vi "CD Init.vi"(8 "Error (in)":errorcluster, 11 "Device Reference":T14 format="%.0x") -> (0 "Error (out)":errorcluster, 1 "Inline Status Channels Refs":T3[](array[typedef]) format="%.0x", 2 "Card Parameters (out)":T25, 3 "RT Inline Data_Data Description_Channels":T17[](array[typedef]) {"Frame Drescriptors"."RT"."Status Channel Ref" format="%.0x"; "Frame Drescriptors"."RT"."Words Block Data Refs"."Data Reference" format="%.0x"; "Frame Drescriptors"."RT"."Timestamp Channel Data Reference" format="%.0x"; "Frame Drescriptors"."BC"."Status Channel Refs" format="%.0x"; "Frame Drescriptors"."BC"."param block data refs"."Data Reference" format="%.0x"; "Frame Drescriptors"."BC"."Timestamp Channel Data Reference" format="%.0x"}, 6 "RT Async Data":T1 {"Map (MC Tx)"."Word Data Reference" format="%.0x"; "Map (MC Rx)"."Channel Data Reference" format="%.0x"; "Map (RT Command Channels)"."RT Command Channel Ref" format="%.0x"; "MAP (BC Acyclic Messages Trigger)"."Acyclic Message Trigger Channel Ref" format="%.0x"; "Map (Bc Command Channels)"."BC Command Channel Ref" format="%.0x"; "Map (RT to ..)"."Word Data Reference" format="%.0x"; "Map (BC to RT)"."Channel Data Reference" format="%.0x"})   [LabVIEW 2020, in "Ballard MIL-1553 Engine.lvlib"]
doc: "This VI reads all properties, creates different Maps (Tx) and initializes the Core of the board using XML file. Initialization is done here because Rx part is done Inline and Tx part asynchronously."
uses:
  Ballard MIL-1553 Engine.lvlib
  <vilib>/NI VeriStand/Custom Device API/Custom Device Item Ref.ctl
  Controls/Card Parameters.ctl
  Shared/Controls and Global/Initialization Method.ctl
  Controls/RT Inline Data_Data Description_Channel.ctl
  Controls/RT Inline Frame Descriptor.ctl
  Controls/RT Inline Frame Descriptor_BC.ctl
  <vilib>/NI VeriStand/Custom Device API/Data Reference.ctl
  <vilib>/NI VeriStand/Custom Device API/Block Data Reference.ctl
  Shared/EncodeDecode/_typedefs/parameter_config_type.ctl
  Shared/EncodeDecode/_typedefs/parameter_config_type_type.ctl
  Shared/EncodeDecode/_typedefs/parameter_config_encoding_type.ctl
  Controls/RT Inline Frame Descriptor_RT.ctl
  Shared/Controls and Global/RT CWD2.ctl
  Shared/Controls and Global/RT CWD1.ctl
  Shared/Controls and Global/RT messageType.ctl
  Controls/RT Async Data.ctl
  Controls/RT Async_Map BC2RT.ctl
  Controls/RT Async_Map_Type.ctl
  Controls/RT Async_Raw Values.ctl
  Controls/RT Async_Raw Values to Messages Index_Association.ctl
  Controls/Asynchronous - Parameter map_type.ctl
  Controls/RT Async_Map RT2BC.ctl
  Controls/RT Async_Map RTs Status.ctl
  Controls/RT Async_Map BC Command Channels.ctl
  Controls/RT Async_Map BC Acyclic Messages Trigger.ctl
  Controls/RT Async_Map RT Command Channels.ctl
  Controls/RT Init States.ctl
  Shared/Controls and Global/Compiled.Settings.ctl
  Shared/Controls and Global/RT Channel.ctl
  Shared/Controls and Global/RT BC.ctl
  Shared/Controls and Global/RT Message.ctl
  Shared/Controls and Global/RT Remote Terminal.ctl
  Shared/Controls and Global/RT Remote Terminal_rtMode.ctl
  Shared/Controls and Global/RT Remote Terminal_RT subAddress.ctl
  Shared/Controls and Global/RT Remote Terminal_RT direction.ctl
  Shared/Controls and Global/RT Remote Terminal_RT Mode Code.ctl
  a0ee2a4f-e665-4580-bc02-68e9c6553bf0.vi
  abe306a3-0000-4c3f-84a0-3b77fc310cf4.vi
  Shared/Controls and Global/Global.vi
  <vilib>/NI VeriStand/Custom Device API/Get Item Property (I32).vi
  <vilib>/NI VeriStand/Custom Device API/Get Item Property (U16).vi
  <vilib>/NI VeriStand/Custom Device API/Get Item Property (Variant).vi
  <vilib>/JDP Science/JSONtext/Variant to JSON Text.vi
  <vilib>/NI VeriStand/Custom Device API/Custom Device API.lvlib
  <vilib>/NI VeriStand/Custom Device Tools/Custom Device Utility Library/Custom Device Utility Library.lvlib
  Shared/Ballard 1553 Shared.lvlib
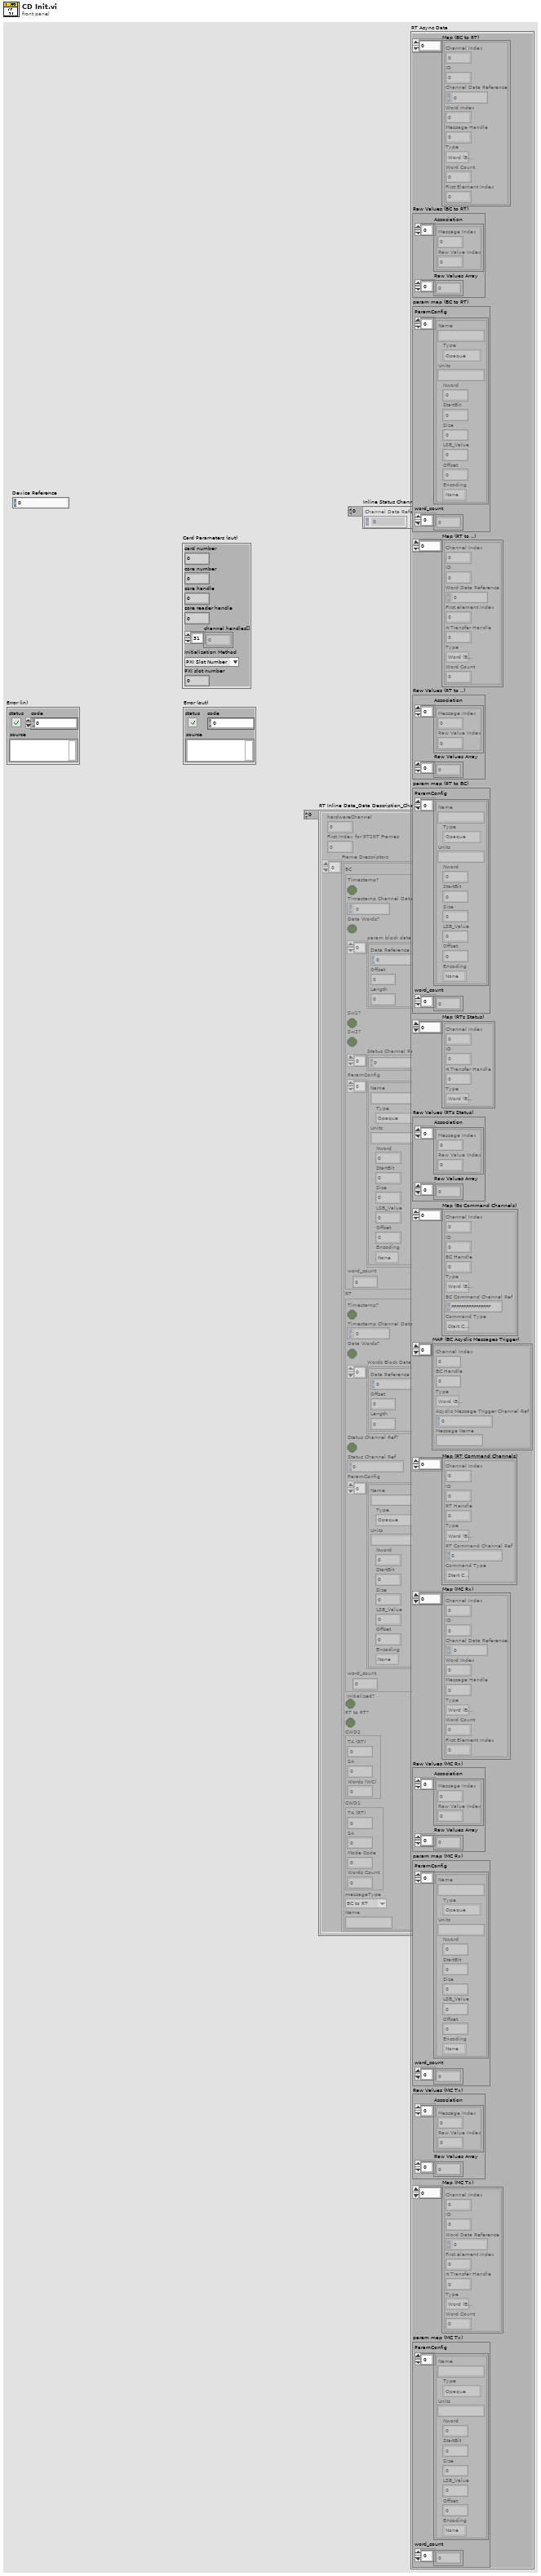
[diagram p1: front panel]
types:
  T1 = typedef "Ballard MIL-1553 Engine.lvlib/RT Async Data.ctl" = cluster{"Map (BC to RT)":T2[], "Raw Values (BC to RT)":T5, "param map (BC to RT)":T7, "Map (RT to ..)":T11[], "Raw Values (RT to ..)":T5, "param map (RT to BC)":T7, "Map (RTs Status)":T12[], "Raw Values (RTs Status)":T5, "Map (Bc Command Channels)":T13[], "MAP (BC Acyclic Messages Trigger)":T15[], "Map (RT Command Channels)":T16[], "Map (MC Rx)":T2[], "Raw Values (MC Rx)":T5, "param map (MC Rx)":T7, "Raw Values (MC Tx)":T5, "Map (MC Tx)":T11[], "param map (MC Tx)":T7}
  T2 = typedef "Ballard MIL-1553 Engine.lvlib/RT Async_Map BC2RT.ctl" = cluster{"Channel Index":i32, "ID":i32, "Channel Data Reference":T3, "Word Index":i32, "Message Handle":u64, "Type":T4, "Word Count":i32, "First Element Index":i32}
  T3 = typedef "Custom Device API.lvlib/Data Reference.ctl" = i32
  T4 = typedef "Ballard MIL-1553 Engine.lvlib/RT Async_Map_Type.ctl" = enum16{"Word (BC to RT)", "Word (MC (Rx))", "Acyclic Message Trigger", "Word (RT to ..)", "Word (RT to RT)", "Word (MC (Tx))", "RT Status", "BC Commands", "RT Commands"}
  T5 = typedef "Ballard MIL-1553 Engine.lvlib/RT Async_Raw Values.ctl" = cluster{"Association":T6[], "Raw Values Array":u16[]}
  T6 = typedef "Ballard MIL-1553 Engine.lvlib/RT Async_Raw Values to Messages Index_Association.ctl" = cluster{"Message Index":i32, "Raw Value Index":i32}
  T7 = typedef "Ballard MIL-1553 Engine.lvlib/Asynchronous - Parameter map_type.ctl" = cluster{"ParamConfig":T8[], "word_count":u8[]}
  T8 = typedef "parameter_config_type.ctl" = cluster{"Name":string, "Type":T9, "Units":string, "Nword":i32, "StartBit":i32, "Size":i32, "LSB_Value":i32, "Offset":i32, "Encoding":T10}
  T9 = typedef "parameter_config_type_type.ctl" = enum16{"Opaque", "Enum", "Float", "Integer", "Bcd", "Bool"}
  T10 = typedef "parameter_config_encoding_type.ctl" = enum16{"None", "2-complement", "Unsigned"}
  T11 = typedef "Ballard MIL-1553 Engine.lvlib/RT Async_Map RT2BC.ctl" = cluster{"Channel Index":i32, "ID":i32, "Word Data Reference":T3, "First element Index":i32, "rt Transfer Handle":u64, "Type":T4, "Word Count":i32}
  T12 = typedef "Ballard MIL-1553 Engine.lvlib/RT Async_Map RTs Status.ctl" = cluster{"Channel Index":i32, "ID":i32, "rt Transfer Handle":u64, "Type":T4}
  T13 = typedef "Ballard MIL-1553 Engine.lvlib/RT Async_Map BC Command Channels.ctl" = cluster{"Channel Index":i32, "ID":i32, "BC Handle":u64, "Type":T4, "BC Command Channel Ref":T14, "Command Type":enum16{"Start Command", "Stop Command"}}
  T14 = typedef "Custom Device API.lvlib/Custom Device Item Ref.ctl" = u64
  T15 = typedef "Ballard MIL-1553 Engine.lvlib/RT Async_Map BC Acyclic Messages Trigger.ctl" = cluster{"Channel Index":i32, "BC Handle":u64, "Type":T4, "Acyclic Message Trigger Channel Ref":T14, "Message Name":string}
  T16 = typedef "Ballard MIL-1553 Engine.lvlib/RT Async_Map RT Command Channels.ctl" = cluster{"Channel Index":i32, "ID":i32, "RT Handle":u64, "Type":T4, "RT Command Channel Ref":T14, "Command Type":enum16{"Start Command", "Stop Command"}}
  T17 = typedef "Ballard MIL-1553 Engine.lvlib/RT Inline Data_Data Description_Channel.ctl" = cluster{"hardwareChannel":u16, "First Index for RT2RT Frames":i32, "Frame Drescriptors":T18[]}
  T18 = typedef "Ballard MIL-1553 Engine.lvlib/RT Inline Frame Descriptor.ctl" = cluster{"BC":T19, "RT":T21, "Initialized?":bool, "RT to RT?":bool, "CWD2":T22, "CWD1":T23, "messageType":T24, "Name":string}
  T19 = typedef "Ballard MIL-1553 Engine.lvlib/RT Inline Frame Descriptor_BC.ctl" = cluster{"Timestamp?":bool, "Timestamp Channel Data Reference":T3, "Data Words?":bool, "param block data refs":T20[], "Sw1?":bool, "Sw2?":bool, "Status Channel Refs":T14[], "ParamConfig":T8[], "word_count":u8}
  T20 = typedef "Custom Device API.lvlib/Block Data Reference.ctl" = cluster{"Data Reference":T3, "Offset":u64, "Length":u64}
  T21 = typedef "Ballard MIL-1553 Engine.lvlib/RT Inline Frame Descriptor_RT.ctl" = cluster{"Timestamp?":bool, "Timestamp Channel Data Reference":T3, "Data Words?":bool, "Words Block Data Refs":T20[], "Status Channel Ref?":bool, "Status Channel Ref":T14, "ParamConfig":T8[], "word_count":u8}
  T22 = typedef "Ballard 1553 Shared.lvlib/RT CWD2.ctl" = cluster{"TA (RT)":i8, "SA":i8, "Words (WC)":i8}
  T23 = typedef "Ballard 1553 Shared.lvlib/RT CWD1.ctl" = cluster{"TA (RT)":i8, "SA":i8, "Mode Code":i8, "Words Count":i8}
  T24 = typedef "Ballard 1553 Shared.lvlib/RT messageType.ctl" = enum16{"BC to RT", "RT to BC", "RT to RT", "MC (Rx)", "MC (Tx)"}
  T25 = typedef "Ballard MIL-1553 Engine.lvlib/Card Parameters.ctl" = cluster{"card number":i32, "core number":i32, "core handle":u64, "core reader handle":u64, "channel handles[]":u64[], "Initialization Method":T26, "PXI slot number":i32}
  T26 = typedef "Ballard 1553 Shared.lvlib/Initialization Method.ctl" = enum16{"PXI Slot Number", "Card Number"}
  T27 = typedef "Ballard MIL-1553 Engine.lvlib/RT Init States.ctl" = enum16{"Initialization", "Get Card Settings", "Get Channel Count", "Parse Channels", "Ballard-1553 Initialize", "Get Status Channels Reference", "Exit"}
  T28 = typedef "Ballard 1553 Shared.lvlib/Compiled.Settings.ctl" = cluster{"Name":string, "channels":T29[]}
  T29 = typedef "Ballard 1553 Shared.lvlib/RT Channel.ctl" = cluster{"name":string, "hardWare Channel Number":u16, "BC":T30, "RTs":T32[]}
  T30 = typedef "Ballard 1553 Shared.lvlib/RT BC.ctl" = cluster{"ID":i32, "name":string, "Command Channels Refs":T14[], "messages":T31[], "Acyclic Frames Trigger Channels Refs":T14[], "Acyclic Frames Names":string[]}
  T31 = typedef "Ballard 1553 Shared.lvlib/RT Message.ctl" = cluster{"Name":string, "messageType":T24, "CWD1":T23, "CWD2":T22, "Status Channel Data Refs":T3[], "param item refs":T14[], "param Block Data Refs":T20[], "param Values Array":u16[], "Timestamp Channel Data Reference":T3, "ID":i32, "Timestamp?":bool, "Data Words?":bool, "Status Channel Ref?":bool, "ParamConfig":T8[], "word_count":u8}
  T32 = typedef "Ballard 1553 Shared.lvlib/RT Remote Terminal.ctl" = cluster{"ID":i32, "name":string, "RT Address":i32, "rtMode":T33, "Command Channels Refs":T14[], "Status Channel Data Reference":T3, "subAddresses":T34[], "Mode Codes":T36[]}
  T33 = typedef "Ballard 1553 Shared.lvlib/RT Remote Terminal_rtMode.ctl" = enum16{"Simulate", "Monitor", "Disable"}
  T34 = typedef "Ballard 1553 Shared.lvlib/RT Remote Terminal_RT subAddress.ctl" = cluster{"name":string, "subAddress":i8, "direction":T35, "Timestamp Channel Data Reference":T3, "param value array":u16[], "param blocj data refs":T20[], "param item refs":T14[], "ID":i32, "Timestamp?":bool, "Data Words?":bool, "param config":T8[], "word_count":u8}
  T35 = typedef "Ballard 1553 Shared.lvlib/RT Remote Terminal_RT direction.ctl" = enum16{"Tx", "Rx"}
  T36 = typedef "Ballard 1553 Shared.lvlib/RT Remote Terminal_RT Mode Code.ctl" = cluster{"name":string, "direction":T35, "Timestamp Channel Data Reference":T3, "param values array":u16[], "param block data refs":T20[], "param item refs":T14[], "ID":i32, "Timestamp?":bool, "Data Words?":bool, "Code Number":i32, "param config":T8[], "word_count":u8}
  T37 = typedef "Custom Device API.lvlib/Custom Device File Dependency.ctl" = cluster{"Source":T38, "RT Destination":path, "ForceDownload?":bool, "SupportedTarget":T40, "Version":string}
  T38 = typedef "Custom Device API.lvlib/Path Specification.ctl" = cluster{"Path":path, "Type":T39}
  T39 = typedef "Custom Device API.lvlib/Path Type.ctl" = enum16{"Absolute", "To Base", "To Common Data Dir", "To Application Data Dir"}
  T40 = typedef "Custom Device API.lvlib/Custom Device Supported Target.ctl" = enum16{"All", "PharLap", "VxWorks", "Windows", "Linux_32_ARM", "Linux_x64", "PharLap & Windows", "PharLap & VxWorks", "VxWorks & Windows"}
  T41 = typedef "Custom Device API.lvlib/Custom Device Item Info.ctl" = cluster{"Name":string, "Is Channel":bool, "GUID":string, "Is Waveform":bool}
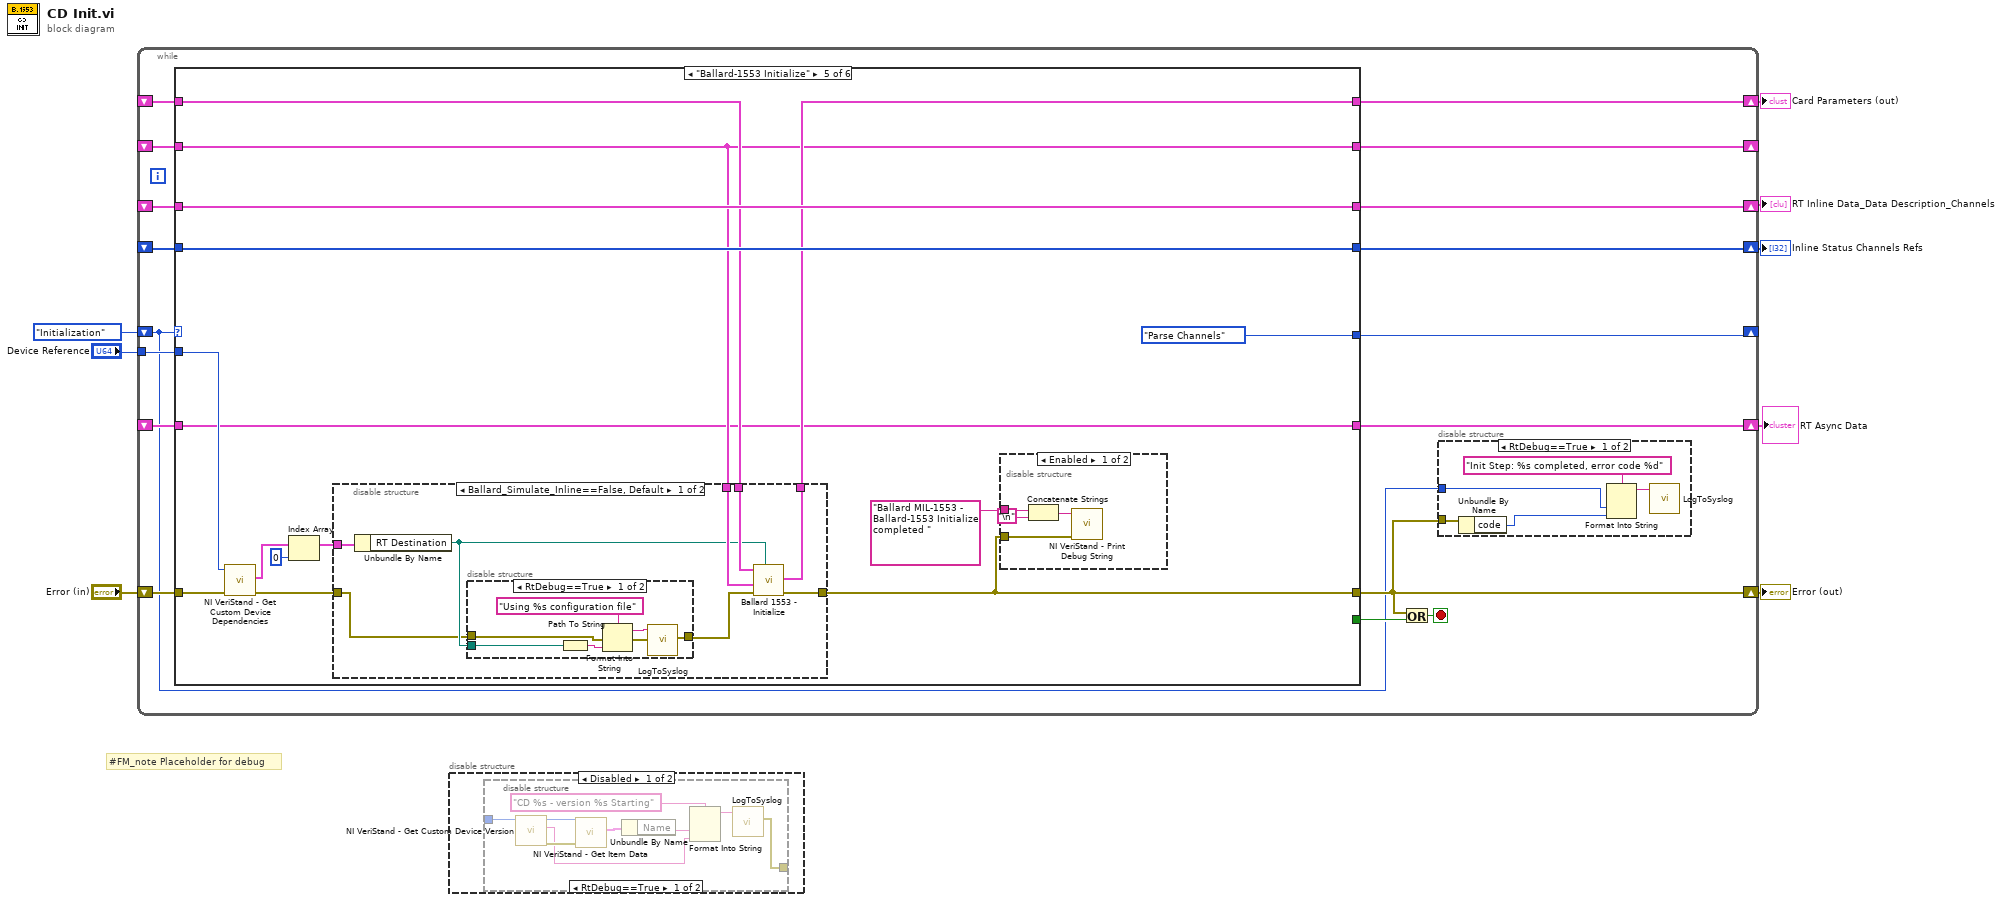
[diagram p0: block diagram]
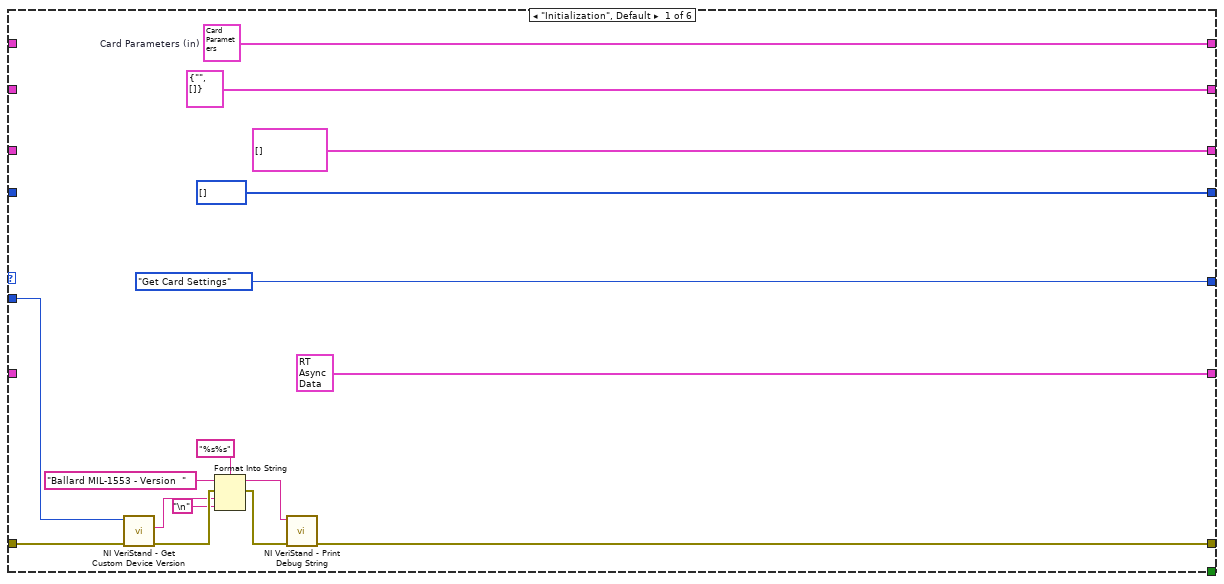
[diagram p5: hidden frame]
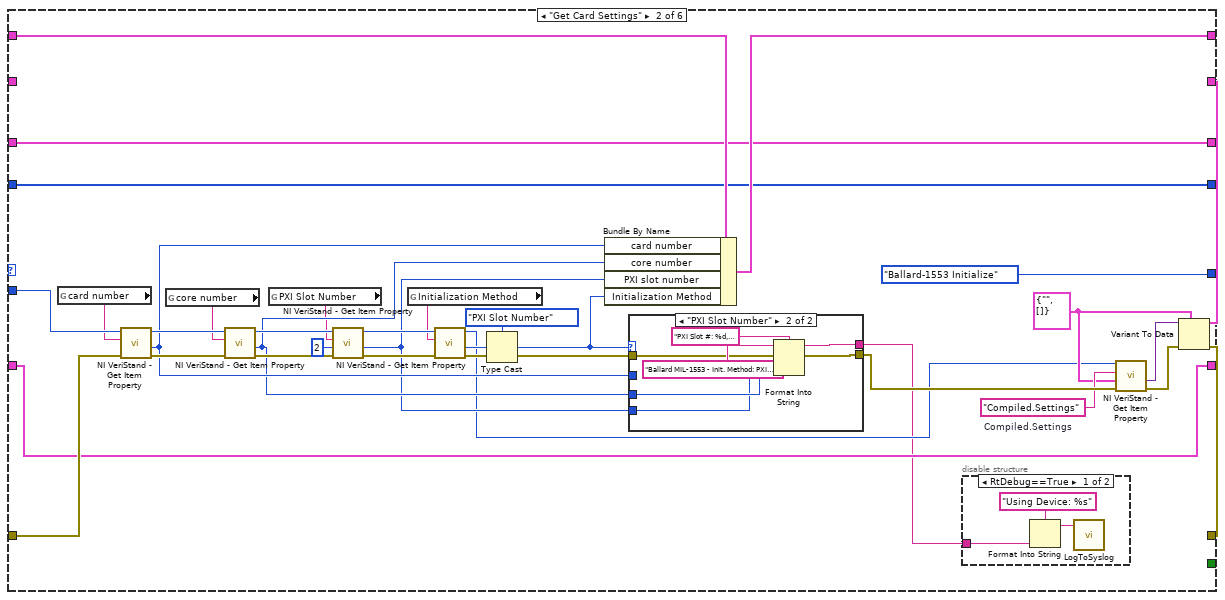
[diagram p6: hidden frame]
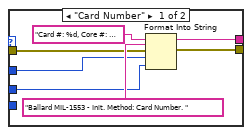
[diagram p8: hidden frame]
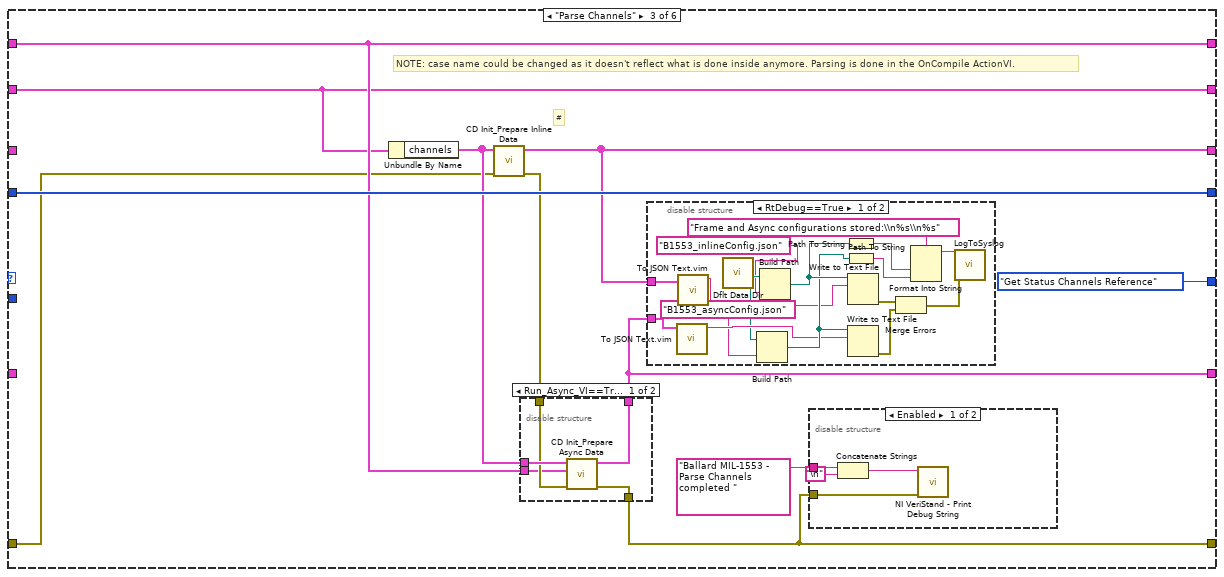
[diagram p9: hidden frame]
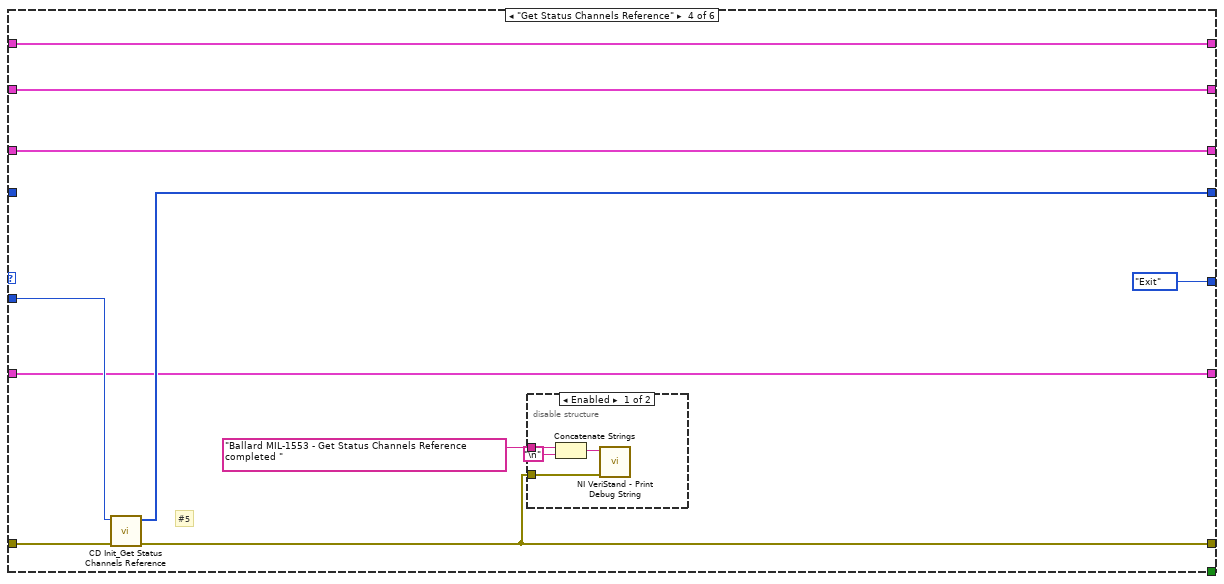
[diagram p13: hidden frame]
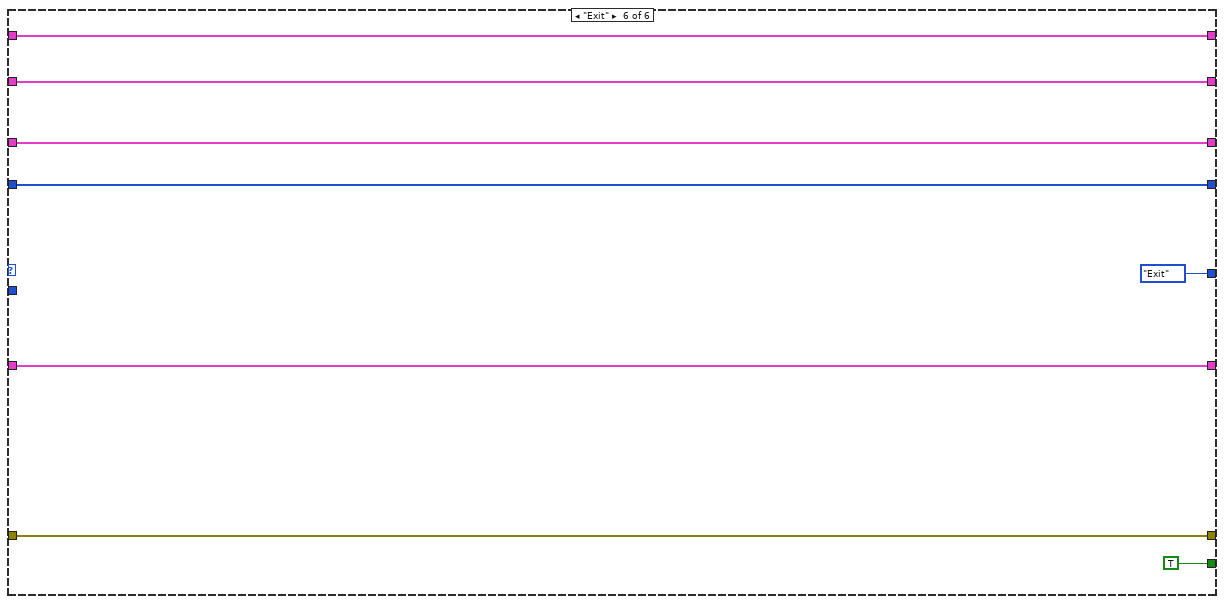
[diagram p18: hidden frame]
diagram:
  # "#FM_note Placeholder for debug"
  n1 = while {
    shift-right: [w11] -> _
    shift-left: RT_Init_States."Initialization" -> [w9]
    tunnel: "Device Reference" -> [w24]
    shift-right: [w20] -> w4
    shift-left: _ -> [w21]
    shift-right: [w19] -> w2
    shift-left: _ -> [w18]
    shift-right: [w17] -> w3
    shift-left: _ -> [w16]
    shift-right: [w10] -> w6
    shift-left: "Error (in)" -> [w25]
    shift-right: [w15] -> _
    shift-left: _ -> [w14]
    shift-right: [w13] -> w1
    shift-left: _ -> [w12]
    stop <- w23 stop-if-true
    n2 = case shown="\"Ballard-1553 Initialize\"" w9 {
      tunnel: w25 -> [w43 w80 w103 w141 w161 w193]
      tunnel: [w41 w49 w101 w136 w150 w193] -> w10
      tunnel: [RT_Init_States."Get Card Settings" RT_Init_States."Ballard-1553 Initialize" RT_Init_States."Get Status Channels Reference" RT_Init_States."Exit" RT_Init_States."Parse Channels" RT_Init_States."Exit"] -> w11
      tunnel: w24 -> [w42 w77 _ w140 w160 _]
      tunnel: [_ _ _ _ _ TRUE] -> w22
      tunnel: w21 -> [_ w76 w106 w142 w154 w190]
      tunnel: [w45 w75 w106 w142 w157 w190] -> w20
      tunnel: [T17[] [] ("RT Inline Data_Data Description_Channels") w74 w100 w145 w159 w189] -> w19
      tunnel: w18 -> [_ w74 _ w145 w159 w189]
      tunnel: [i32[] [] w73 w108 w143 w158 w188] -> w17
      tunnel: w16 -> [_ w73 w108 _ w158 w188]
      tunnel: [T28 {"Name"="", "channels"=[]} ("Compiled.Settings") w48 w104 w139 w153 w187] -> w15
      tunnel: w14 -> [_ _ w104 w139 w153 w187]
      tunnel: [T1 {"Map (BC to RT)"=[], "Raw Values (BC to RT)"={"Association"=[], "Raw Values Array"=[]}, "param map (BC to RT)"={"ParamConfig"=[], "word_count"=[]}, "Map (RT to ..)"=[], "Raw Values (RT to ..)"={"Association"=[], "Raw Values Array"=[]}, "param map (RT to BC)"={"ParamConfig"=[], "word_count"=[]}, "Map (RTs Status)"=[], "Raw Values (RTs Status)"={"Association"=[], "Raw Values Array"=[]}, "Map (Bc Command Channels)"=[], "MAP (BC Acyclic Messages Trigger)"=[], "Map (RT Command Channels)"=[], "Map (MC Rx)"=[], "Raw Values (MC Rx)"={"Association"=[], "Raw Values Array"=[]}, "param map (MC Rx)"={"ParamConfig"=[], "word_count"=[]}, "Raw Values (MC Tx)"={"Association"=[], "Raw Values Array"=[]}, "Map (MC Tx)"=[], "param map (MC Tx)"={"ParamConfig"=[], "word_count"=[]}} ("RT Async Data") w55 w99 w138 w152 w186] -> w13
      tunnel: w12 -> [_ w55 _ w138 w152 w186]
      frame "Initialization", Default {
        w45 = T25 {"card number"=0, "core number"=0, "core handle"=0, "core reader handle"=0, "channel handles[]"=[], "Initialization Method"=enum."PXI Slot Number", "PXI slot number"=0}  # Card Parameters (in)
        n3 = call <vilib>:"NI VeriStand - Get Custom Device Version.vi"("error in (no error)"=w43, "Device Ref in"=w42) -> ("error out"=w40:errorcluster, "Value"=w37:string)  [unwired: 7 in, 1 out]
        n4 = Format Into String(format string="%s%s", initial string="Ballard MIL-1553 - Version  ", error in=w40, w37, "\n") -> (resulting string=w31:string, error out=w39:errorcluster)
        n5 = call <vilib>:"NI VeriStand - Print Debug String.vi"("error in (no error)"=w39, "Message"=w31) -> ("error out"=w41:errorcluster)  [unwired: 9 in]
      }
      frame "Get Card Settings" {
        w52 = "Compiled.Settings"  # Compiled.Settings
        w51 = T28 {"Name"="", "channels"=[]} ("Compiled.Settings")
        n6 = global read "Global.vi" "card number"() -> (w56:string)
        n7 = call-poly <vilib>:"NI VeriStand - Get Item Property.vi"("error in (no error)"=w80, "Property Name"=w56, "Item Ref in"=w77) -> ("error out"=w79:errorcluster, "Value"=w64:i32, "Item Ref out"=w81:T14)  [unwired: 5 in, 1 out]
        n8 = global read "Global.vi" "core number"() -> (w57:string)
        n9 = call-poly <vilib>:"NI VeriStand - Get Item Property.vi"("error in (no error)"=w79, "Property Name"=w57, "Item Ref in"=w81) -> ("error out"=w71:errorcluster, "Value"=w63:i32, "Item Ref out"=w72:T14)  [unwired: 5 in, 1 out]
        n10 = global read "Global.vi" "PXI Slot Number"() -> (w58:string)
        n11 = call-poly <vilib>:"NI VeriStand - Get Item Property.vi"("error in (no error)"=w71, "Default Value"=2, "Property Name"=w58, "Item Ref in"=w72) -> ("error out"=w69:errorcluster, "Value"=w62:i32, "Item Ref out"=w68:T14)  [unwired: 4 in, 1 out]
        n12 = global read "Global.vi" "Initialization Method"() -> (w59:string)
        n13 = call-poly <vilib>:"NI VeriStand - Get Item Property.vi"("error in (no error)"=w69, "Property Name"=w59, "Item Ref in"=w68) -> ("error out"=w61:errorcluster, "Value"=w67:u16, "Item Ref out"=w50:T14)  [unwired: 5 in, 1 out]
        n14 = Type Cast(type=Initialization_Method."PXI Slot Number" ("Initialization Method"), x=w67) -> (*(type *) &x=w65:T26)
        n15 = Bundle By Name(cluster=w76, "card number"=w64, "core number"=w63, "PXI slot number"=w62, "Initialization Method"=w65) -> (w75:T25)
        n16 = case shown="\"PXI Slot Number\"" w65 {
          tunnel: [w91 w98] -> w47
          tunnel: w64 -> [w88 _]
          tunnel: w63 -> [w87 w95]
          tunnel: w62 -> [_ w94]
          tunnel: w61 -> [w86 w93]
          tunnel: [w85 w92] -> w60
          frame "Card Number" {
            n17 = Format Into String(format string="Card #: %d, Core #: %d.", initial string="Ballard MIL-1553 - Init. Method: Card Number. " ("String to write"), error in=w86, w88, w87) -> (resulting string=w91:string, error out=w85:errorcluster)
          }
          frame "PXI Slot Number" {
            n18 = Format Into String(format string="PXI Slot #: %d, Core #: %d.", initial string="Ballard MIL-1553 - Init. Method: PXI Slot Number. " ("String to write"), error in=w93, w94, w95) -> (resulting string=w98:string, error out=w92:errorcluster)
          }
        }
        n19 = disable-structure shown="RtDebug==True" {
          disable-tunnel: w47 -> [w82 _]
          frame condition #0 (active) {
            n20 = Format Into String(format string="Using Device: %s", w82) -> (resulting string=w84:string)  [unwired: 2 in, 1 out]
            n21 = call "LogToSyslog.vi"("message"=w84) -> ()  [unwired: 9 in, 2 out]
          }
          frame condition #1 {
          }
        }
        n22 = call-poly <vilib>:"NI VeriStand - Get Item Property.vi"("error in (no error)"=w60, "Default Value"=w51, "Property Name"=w52, "Item Ref in"=w50) -> ("error out"=w54:errorcluster, "Value"=w53:variant)  [unwired: 4 in, 2 out]
        n23 = Variant To Data(error in=w54, type=w51, Variant=w53) -> (data=w48:T28, error out=w49:errorcluster)
      }
      frame "Parse Channels" {
        # "#"
        # "NOTE: case name could be changed as it doesn't reflect what is done inside anymore. Parsing is done in the OnCompile ActionVI."
        n24 = Unbundle By Name(w104) -> ("channels"=w107:T29[])
        n25 = call "CD Init_Prepare Inline Data.vi"("error in (no error)"=w103, "channels In"=w107) -> ("error out"=w102:errorcluster, "RT Inline Data_Data Description_Channels"=w100:T17[])  [unwired: 8 in]
        n26 = disable-structure shown="Run_Async_VI==True, Default" {
          disable-tunnel: w107 -> [w130 _]
          disable-tunnel: w102 -> [w129 w131]
          disable-tunnel: w106 -> [w128 _]
          disable-tunnel: [w127 _] -> w99
          disable-tunnel: [w126 w131] -> w101
          frame condition #0 (active) {
            n27 = call "CD Init_Prepare Async Data.vi"("error in (no error)"=w129, "Card Parameters (in)"=w128, "Channels In"=w130) -> ("error out"=w126:errorcluster, "RT Async Data"=w127:T1)  [unwired: 7 in]
          }
          frame condition #1 {
          }
        }
        n28 = disable-structure shown="RtDebug==True" {
          disable-tunnel: w100 -> [w117 _]
          disable-tunnel: w99 -> [w116 _]
          frame condition #0 (active) {
            n29 = call "To JSON Text.vim"("Anything"=w116) -> ("<JSON>"=w115:string)  [unwired: 9 in, 1 out]
            n30 = call "To JSON Text.vim"("Anything"=w117) -> ("<JSON>"=w114:string)  [unwired: 9 in, 1 out]
            n31 = call <vilib>:"Dflt Data Dir.vi"() -> ("App:Default Data Directory"=w112:path)
            n32 = Build Path(base path=w112, name or relative path="B1553_asyncConfig.json" ("format string")) -> (appended path=w118:path)
            n33 = Build Path(base path=w112, name or relative path="B1553_inlineConfig.json" ("format string")) -> (appended path=w119:path)
            n34 = Path To String(path=w119) -> (string=w122:string)
            n35 = Path To String(path=w118) -> (string=w120:string)
            n36 = Write to Text File(file (use dialog)=w119, text=w114) -> (error out=w125:errorcluster)  [unwired: 2 in, 2 out]
            n37 = Write to Text File(file (use dialog)=w118, text=w115) -> (error out=w124:errorcluster)  [unwired: 2 in, 2 out]
            n38 = Merge Errors(w125, w124) -> (w123:errorcluster)
            n39 = Format Into String(format string="Frame and Async configurations stored:\\n%s\\n%s", w122, w120) -> (resulting string=w113:string)  [unwired: 2 in, 1 out]
            n40 = call "LogToSyslog.vi"("error in (no error)"=w123, "message"=w113) -> ()  [unwired: 8 in, 2 out]
          }
          frame condition #1 {
          }
        }
        n41 = disable-structure shown="Enabled" {
          disable-tunnel: w101 -> [w134 _]
          disable-tunnel: "Ballard MIL-1553 - Parse Channels completed " -> [w133 _]
          frame Enabled {
            n42 = Concatenate Strings(w133, "\n") -> (w132:string)
            n43 = call <vilib>:"NI VeriStand - Print Debug String.vi"("error in (no error)"=w134, "Message"=w132) -> ()  [unwired: 9 in, 1 out]
          }
          frame Disabled {
          }
        }
      }
      frame "Get Status Channels Reference" {
        # "#5"
        n44 = call "CD Init_Get Status Channels Reference.vi"("error in (no error)"=w141, "Device Reference"=w140) -> ("error out"=w136:errorcluster, "Array"=w143:T3[])  [unwired: 8 in]
        n45 = disable-structure shown="Enabled" {
          disable-tunnel: w136 -> [w148 _]
          disable-tunnel: "Ballard MIL-1553 - Get Status Channels Reference completed " -> [w147 _]
          frame Enabled {
            n46 = Concatenate Strings(w147, "\n") -> (w146:string)
            n47 = call <vilib>:"NI VeriStand - Print Debug String.vi"("error in (no error)"=w148, "Message"=w146) -> ()  [unwired: 9 in, 1 out]
          }
          frame Disabled {
          }
        }
      }
      frame "Ballard-1553 Initialize" {
        n48 = call <vilib>:"NI VeriStand - Get Custom Device Dependencies.vi"("error in (no error)"=w161, "Device Ref in"=w160) -> ("error out"=w155:errorcluster, "Dependencies"=w163:T37[])  [unwired: 7 in, 1 out]
        n49 = Index Array(array=w163, index=0) -> (element=w162:T37)
        n50 = disable-structure shown="Ballard_Simulate_Inline==False, Default" {
          disable-tunnel: w162 -> [w172 _]
          disable-tunnel: [w171 w180] -> w157
          disable-tunnel: w155 -> [w166 w181]
          disable-tunnel: w154 -> [w170 w180]
          disable-tunnel: w153 -> [w169 _]
          disable-tunnel: [w168 w181] -> w150
          frame condition #0 (active) {
            n51 = Unbundle By Name(w172) -> ("RT Destination"=w167:path)
            n52 = disable-structure shown="RtDebug==True" {
              disable-tunnel: w167 -> [w178 _]
              disable-tunnel: w166 -> [w175 _]
              disable-tunnel: [w173 _] -> w165
              frame condition #0 (active) {
                n53 = Path To String(path=w178) -> (string=w179:string)
                n54 = Format Into String(format string="Using %s configuration file", error in=w175, w179) -> (resulting string=w176:string, error out=w174:errorcluster)  [unwired: 1 in]
                n55 = call "LogToSyslog.vi"("error in (no error)"=w174, "message"=w176) -> ("error out"=w173:errorcluster)  [unwired: 8 in, 1 out]
              }
              frame condition #1 {
              }
            }
            n56 = call "Ballard 1553 - Initialize.vi"("RT Config Filepath"=w167, "Error (in)"=w165, "Compiled.Settings"=w169, "Card Parameters (in)"=w170) -> ("Error (out)"=w168:errorcluster, "Card Parameters (out)"=w171:T25)  [unwired: 6 in]
          }
          frame condition #1 {
          }
        }
        n57 = disable-structure shown="Enabled" {
          disable-tunnel: w150 -> [w184 _]
          disable-tunnel: "Ballard MIL-1553 - Ballard-1553 Initialize completed " -> [w183 _]
          frame Enabled {
            n58 = Concatenate Strings(w183, "\n") -> (w182:string)
            n59 = call <vilib>:"NI VeriStand - Print Debug String.vi"("error in (no error)"=w184, "Message"=w182) -> ()  [unwired: 9 in, 1 out]
          }
          frame Disabled {
          }
        }
      }
      frame "Exit" {
      }
    }
    n60 = Or(x=w10, y=w22) -> (x .or. y?=w23:bool)
    n61 = disable-structure shown="RtDebug==True" {
      disable-tunnel: w9 -> [w26 _]
      disable-tunnel: w10 -> [w28 _]
      frame condition #0 (active) {
        n62 = Unbundle By Name(w28) -> ("code"=w27:i32)
        n63 = Format Into String(format string="Init Step: %s completed, error code %d", w26, w27) -> (resulting string=w30:string)  [unwired: 2 in, 1 out]
        n64 = call "LogToSyslog.vi"("message"=w30) -> ()  [unwired: 9 in, 2 out]
      }
      frame condition #1 {
      }
    }
  }
  "Error (out)" <- w6
  "Card Parameters (out)" <- w4
  "RT Inline Data_Data Description_Channels" <- w2
  "Inline Status Channels Refs" <- w3
  "RT Async Data" <- w1
  n65 = disable-structure shown="Disabled" {
    frame Disabled {
      n66 = disable-structure shown="RtDebug==True" {
        disable-tunnel: _ -> [w202 _]
        disable-tunnel: [w196 _] -> _
        frame condition #0 (active) {
          n67 = call <vilib>:"NI VeriStand - Get Custom Device Version.vi"("Device Ref in"=w202) -> ("error out"=w200:errorcluster, "Value"=w194:string, "Device Ref out"=w201:T14)  [unwired: 8 in]
          n68 = call <vilib>:"NI VeriStand - Get Item Data.vi"("error in (no error)"=w200, "Item Ref in"=w201) -> ("Item Info"=w199:T41)  [unwired: 9 out]
          n69 = Unbundle By Name(w199) -> ("Name"=w195:string)
          n70 = Format Into String(format string="CD %s - version %s Starting", w195, w194) -> (resulting string=w198:string)  [unwired: 2 in, 1 out]
          n71 = call "LogToSyslog.vi"("message"=w198) -> ("error out"=w196:errorcluster)  [unwired: 9 in, 1 out]
        }
        frame condition #1 {
        }
      }
    }
    frame Enabled {
    }
  }
